vi "GetDataForExcel.MatchRegExp.vi"(7 "Journal":u16, 8 "error in":errorcluster, 11 "path":path) -> (0 "error out":errorcluster, 1 "Active":string[](array[string]), 2 "Normal":string[](array[string]), 3 "path out":path)   [LabVIEW 2013, in "main.lvlib"]
uses:
  main.lvlib
  Controls/Enum Variables.ctl
  <vilib>/regexp/Match Regular Expression.xnode
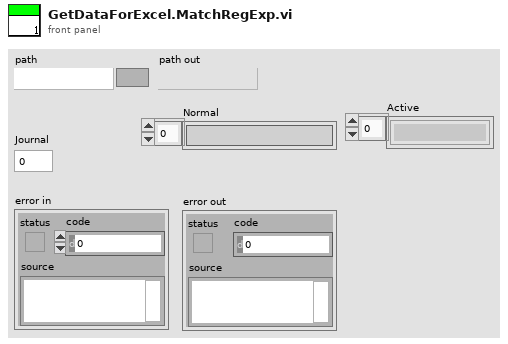
[diagram p1: front panel]
types:
  T1 = typedef "main.lvlib/Enum Variables.ctl" = enum16{"SetAcqFilter", "GetAcqFilter", "Set Filter", "Get Filter", "Set Height", "Get Height", "Set Recorded Height", "Get Recorded Height", "Set Blue Pressure", "Get Blue Pressure", "Set Red Pressure", "Get Red Pressure", "Init", "Reset Pressure", "Set Red Cursors", "Get Red Cursors", "Set Blue Cursors", "Get Blue Cursors", "Set Language", "Get Language", "Set Active Graphs", "Get ActiveGraphs", "Set Method", "Get Method", "Set Encryption", "Get Encryption", "Set ExcelVersion", "Get ExcelVersion", "Set DICOM Avail", "Get DICOM Avail", "Set DICOM Encode", "Get DICOM Encode", "Set JournalExport", "Get JournalExport", "Set Sequence", "Get Sequence", "Set DAQ Connected", "Get DAQ Connected", "Set Current Graph", "Get Current Graph", "Set General Settings", "Get Hyphenation", "Set Arm Calc Method", "Get Arm Calc Method", "Set Dicom Tags", "Get Dicom Tags", "Set BT Serial", "Get BT Serial", "Set BT Accepted Serials", "Get BT Accepted Serials", "Get BT License", "Set BT License"}
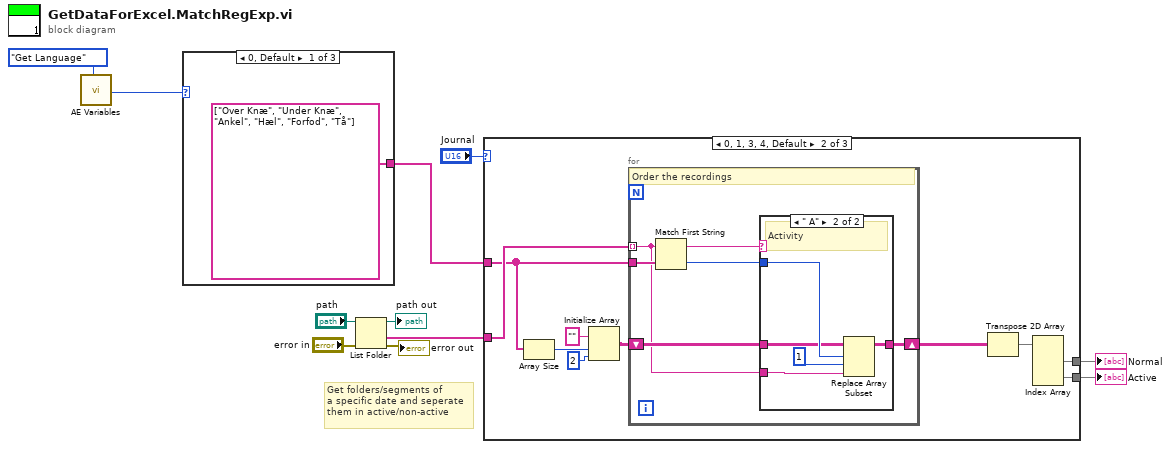
[diagram p0: block diagram]
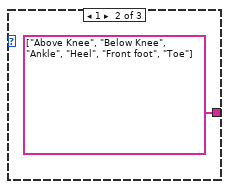
[diagram p2: hidden frame]
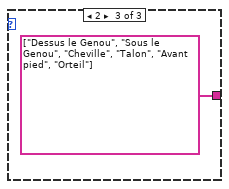
[diagram p3: hidden frame]
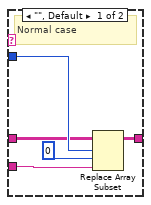
[diagram p5: hidden frame]
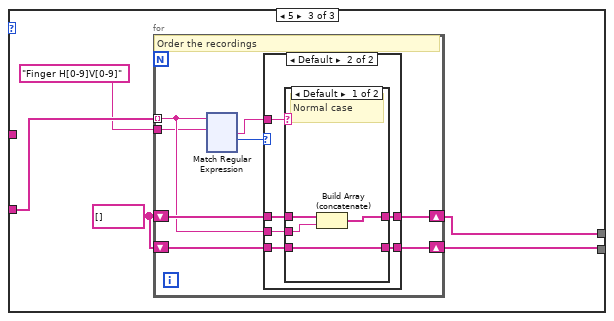
[diagram p6: hidden frame]
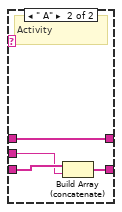
[diagram p8: hidden frame]
diagram:
  # "Get folders/segments of \na specific date and seperate\nthem in active/non-active"
  n1 = call "AE Variables.vi"("Action"=Enum_Variables."Get Language") -> ("RingOut"=w3:u16)  [unwired: 11 in, 7 out]
  n2 = case shown="0, Default" w3 {
    tunnel: [string[] ["Over Knæ", "Under Knæ", "Ankel", "Hæl", "Forfod", "Tå"] string[] ["Above Knee", "Below Knee", "Ankle", "Heel", "Front foot", "Toe"] string[] ["Dessus le Genou", "Sous le Genou", "Cheville", "Talon", "Avant pied", "Orteil"]] -> w5
    frame 0, Default {
    }
    frame 1 {
    }
    frame 2 {
    }
  }
  n3 = List Folder(path="path", error in="error in") -> (path out=→"path out":path, folder names=w10:string[], error out=→"error out":errorcluster)  [unwired: 2 in, 1 out]
  n4 = case shown="0, 1, 3, 4, Default" "Journal" {
    tunnel: w10 -> [w15 w25 w46]
    tunnel: [w15 w17 w44] -> w2
    tunnel: w5 -> [_ w23 _]
    tunnel: [_ w16 w43] -> w1
    frame 2 {
    }
    frame 0, 1, 3, 4, Default {
      n5 = Array Size(array=w23) -> (size(s)=w24:i32)
      n6 = Initialize Array("", w24, 2 ("dimension size")) -> (w21:string[][])
      n7 = for {
        tunnel: w25 -> [w27] mode=indexing
        tunnel: w23 -> [w30]
        shift-right: [w26] -> w19
        shift-left: w21 -> [w29]
        # "Order the recordings"
        n8 = Match First String(2:w30, 3:w27) -> (0:w31:i32, 1:w28:string)
        n9 = case shown="\" A\"" w28 {
          tunnel: w31 -> [w36 w41]
          tunnel: w29 -> [w34 w39]
          tunnel: w27 -> [w32 w37]
          tunnel: [w35 w40] -> w26
          frame "", Default {
            # "Normal case"
            n10 = Replace Array Subset(array=w34, new element=w32, index (row)=w36, index (col)=0 ("disabled index (col)")) -> (w35:string[][])
          }
          frame " A" {
            # "Activity"
            n11 = Replace Array Subset(array=w39, new element=w37, index (row)=w41, index (col)=1 ("disabled index (col)")) -> (w40:string[][])
          }
        }
      }
      n12 = Transpose 2D Array(2D array=w19) -> (transposed array=w18:string[][])
      n13 = Index Array(array=w18) -> (element #1=w17:string[], element #2=w16:string[])  [unwired: 4 in]
    }
    frame 5 {
      w42 = string[] []
      n14 = for {
        tunnel: w46 -> [w52] mode=indexing
        shift-right: [w53] -> w44
        shift-left: w42 -> [w54]
        tunnel: "Finger H[0-9]V[0-9]" -> [w51]
        shift-right: [w48] -> w43
        shift-left: w42 -> [w49]
        # "Order the recordings"
        n15 = xnode "Match Regular Expression"("input string"=w52, "regular expression"=w51) -> ("after match"=w50:string, "offset past match"=w47:i32)  [unwired: 4 in, 3 out]
        n16 = case shown="Default" w47 {
          tunnel: w54 -> [w56 w62]
          tunnel: [w56 w61] -> w53
          tunnel: w52 -> [_ w60]
          tunnel: w50 -> [_ w59]
          tunnel: w49 -> [w55 w58]
          tunnel: [w55 w57] -> w48
          frame -1 {
          }
          frame Default {
            n17 = case shown="Default" w59 {
              tunnel: w62 -> [w66 w70]
              tunnel: w60 -> [w64 w68]
              tunnel: [w65 w70] -> w61
              tunnel: w58 -> [w63 w69]
              tunnel: [w63 w67] -> w57
              frame Default {
                # "Normal case"
                n18 = Build Array (concatenate)(w66, w64) -> (w65:string[])
              }
              frame " A" {
                # "Activity"
                n19 = Build Array (concatenate)(w69, w68) -> (w67:string[])
              }
            }
          }
        }
      }
    }
  }
  "Normal" <- w2
  "Active" <- w1
